vi "[Version] - Get Application Main.vi"() -> (0 "Version":string)   [LabVIEW 2020]
uses:
  TypeDefs/ENUM_Application Files List.ctl
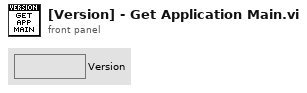
[diagram p1: front panel]
types:
  T1 = typedef "ENUM_Application Files List.ctl" = enum16{"<Example> Folder", "<Example>.txt", "<Example>.csv", "Application.exe"}
  T2 = enum32{"invalid app kind", "Development System", "Run Time System", "Student Edition", "Embedded LabVIEW", "Evaluation", "Custom"}
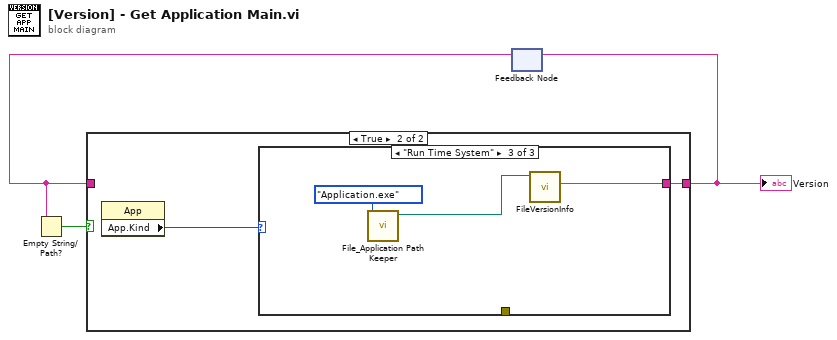
[diagram p0: block diagram]
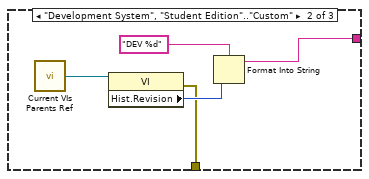
[diagram p4: hidden frame]
diagram:
  n1 = feedback #1() -> (w2:string)  [unwired: 1 in]
  n2 = Empty String/Path?(string/path=w2) -> (empty?=w1:bool)
  n3 = case shown="True" w1 {
    tunnel: [w4 w6] -> w3
    tunnel: w2 -> [w4 _]
    frame False {
    }
    frame True {
      n4 = property class="App"() -> ("App.Kind"=w5:T2)  [unwired: 2 in, 2 out]
      n5 = case shown="\"Run Time System\"" w5 {
        tunnel: [_ w9 w14] -> w6
        tunnel: [_ w7 _] -> _
        frame "invalid app kind" {
        }
        frame "Development System", "Student Edition".."Custom" {
          n6 = call "Current VIs Parents Ref.vi"() -> ("Calling VI's reference"=w8:refnum<vi>)  [unwired: 2 in]
          n7 = property class="VI"(reference=w8) -> (error out=w7:errorcluster, "Hist.Revision"=w11:u32)  [unwired: 1 in, 1 out]
          n8 = Format Into String(format string="DEV %d", w11) -> (resulting string=w9:string)  [unwired: 2 in, 1 out]
        }
        frame "Run Time System" {
          n9 = call "File_Application Path Keeper.vi"("Application  Files Select"=ENUM_Application_Files_List."Application.exe" ("File Keeper Files")) -> ("Path Out"=w12:path)  [unwired: 8 in, 2 out]
          n10 = call <vilib>:"FileVersionInfo.vi"("Application Path in"=w12) -> ("File Version Info"=w14:string)  [unwired: 7 in, 3 out]
        }
      }
    }
  }
  "Version" <- w3
  n11 = feedback-in #1(w3) -> ()
